vi "PMX_Device.vi"(8 "Error in":errorcluster, 9 "Port":i32=55000, 10 "IPAddress":string) -> (0 "Error out":errorcluster, 3 "Device":refnum<k24>)   [LabVIEW 2016]
doc: "Generates a new PMX device.\n\nIPAddress: IPAddress of the device you want to connect with\nPort: Port of the device you want to connect with (default port is 55000)"
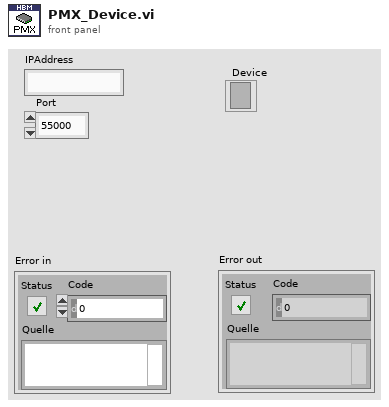
[diagram p1: front panel]
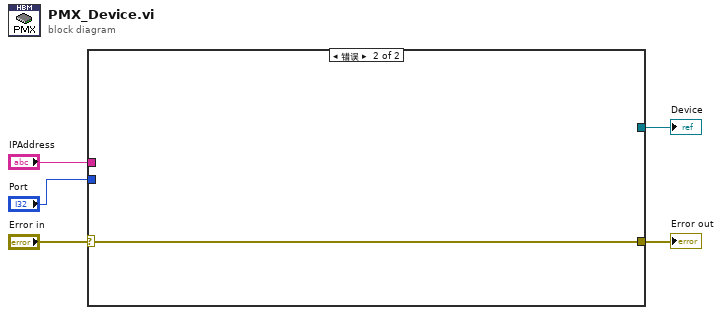
[diagram p0: block diagram]
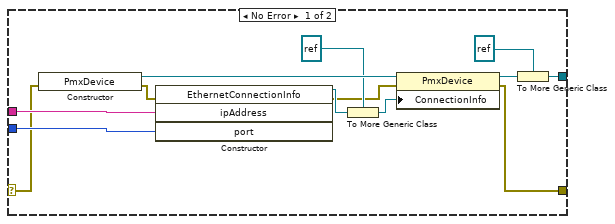
[diagram p2: hidden frame]
diagram:
  n1 = case shown="错误" "Error in" {
    selector: "Error in" -> [w10 w19]
    tunnel: "IPAddress" -> [w18 _]
    tunnel: "Port" -> [w17 _]
    tunnel: [w6 w19] -> w2
    tunnel: [w12 _] -> w1
    frame No Error {
      n2 = constructor class="PmxDevice"(error in=w10) -> (reference out=w14:refnum<k24>, error out=w15:errorcluster)  [unwired: 2 in, 1 out]
      n3 = constructor class="EthernetConnectionInfo"(error in=w15, "ipAddress"=w18, "port"=w17) -> (reference out=w16:refnum<k24>, error out=w8:errorcluster)  [unwired: 2 in, 3 out]
      n4 = To More Generic Class(target class=refnum<k24> refnum (".NET (Referenz)"), reference=w16) -> (generic class reference=w13:refnum<k24>)
      n5 = property on="Eigenschaftsknoten" class="PmxDevice"(reference=w14, error in=w8, "ConnectionInfo"=w13) -> (reference out=w11:refnum<k24>, error out=w6:errorcluster)
      n6 = To More Generic Class(target class=refnum<k24> refnum (".NET (Referenz)"), reference=w11) -> (generic class reference=w12:refnum<k24>)
    }
    frame Error {
    }
  }
  "Error out" <- w2
  "Device" <- w1
